vi "GKÇ-2_Deneme_Veri_Yaz.vi"() -> ()   [LabVIEW 2014]
panel:
  in  "stop":bool
  in  "Array":dbl[](array[numeric])=[0.0, 1.0, 2.0, 0.0, 5.0, 0.0, 0.0, 8.0]
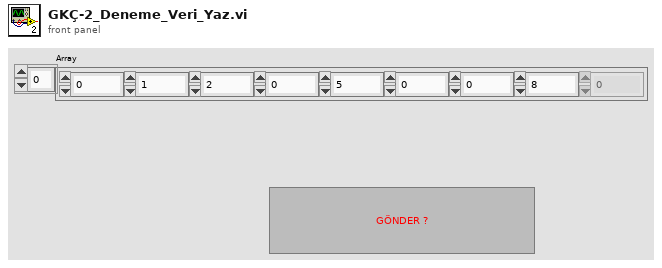
[diagram p1: front panel]
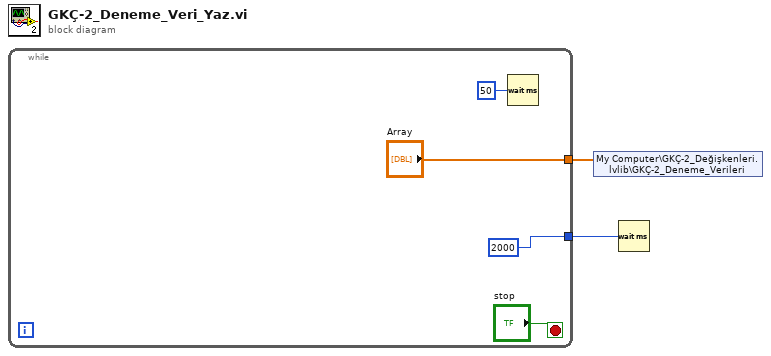
[diagram p0: block diagram]
diagram:
  n1 = while {
    tunnel: ["Array"] -> w2
    tunnel: [u32 2000 ("milliseconds to wait")] -> w1
    stop <- "stop" stop-if-true
    n2 = Wait (ms)(milliseconds to wait=u32 50) -> ()  [unwired: 1 out]
  }
  n3 = shared-variable "My Computer\\GKÇ-2_Değişkenleri.lvlib\\GKÇ-2_Deneme_Verileri"(w2) -> ()  [unwired: 1 in, 1 out]
  n4 = Wait (ms)(milliseconds to wait=w1) -> ()  [unwired: 1 out]
